vi "App Directory Folder and File Handler.vi"(8 "error in":errorcluster) -> (0 "error out":errorcluster, 1 "Setup Files Folder":path, 3 "Report Template Folder":path, 4 "Report Folder":path)   [LabVIEW 2018, in "File IO.lvlib"]
uses:
  File IO.lvlib
  <vilib>/Utility/sysdir.llb/System Directory Type.ctl
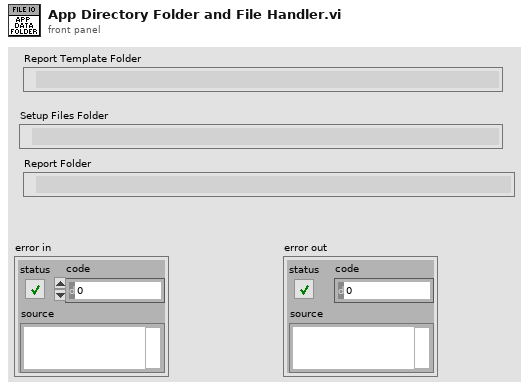
[diagram p1: front panel]
types:
  T1 = typedef "System Directory Type.ctl" = i32
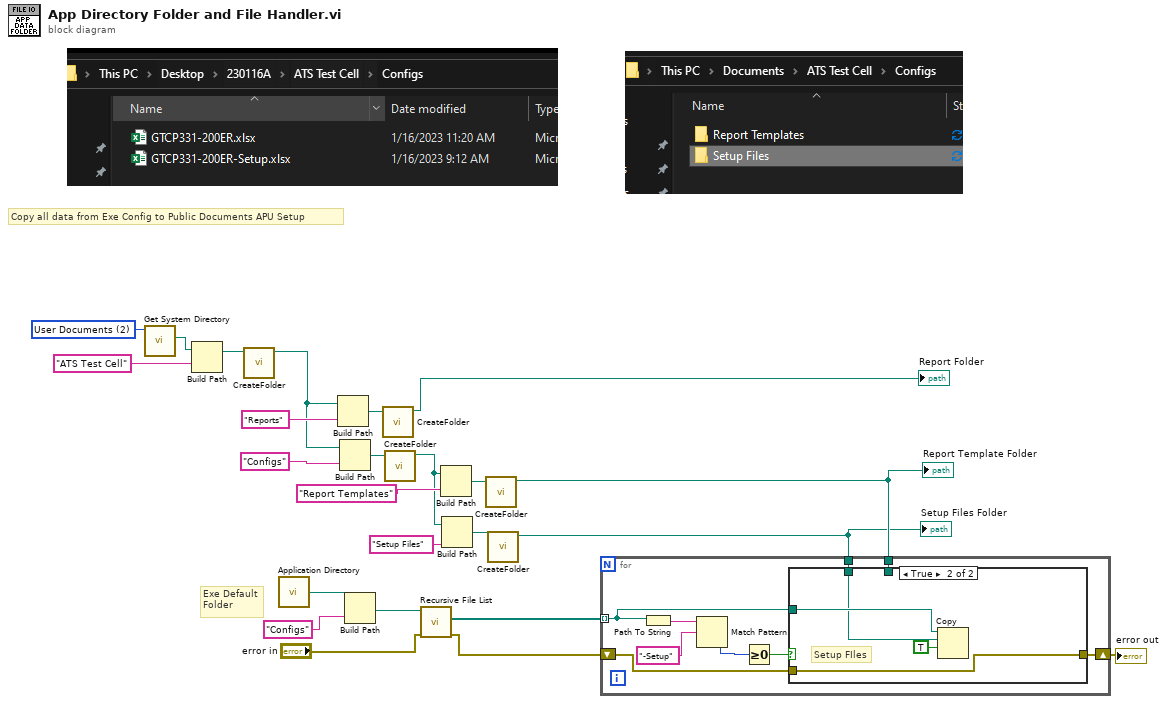
[diagram p0: block diagram]
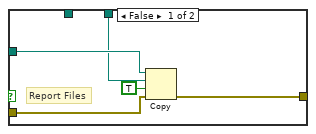
[diagram p2: hidden frame]
diagram:
  w24 = T1 2 items=["User Home"=0, "User Desktop"=1, "User Documents"=2, "User Application Data"=3, "User Preferences"=4, "User Temporary"=5, "Public Documents"=6, "Public Application Data"=7, "Public Preferences"=8, "Public Cache"=13, "System Core Libraries"=9, "System Installed Libraries"=10, "Application Files"=11, "Boot Volume Root"=12] ("system directory type")
  # "Exe Default\nFolder"
  # "Copy all data from Exe Config to Public Documents APU Setup"
  n1 = call <vilib>:"Get System Directory.vi"("system directory type"=w24) -> ("system directory"=w23:path)  [unwired: 10 in]
  n2 = Build Path(base path=w23, name or relative path="ATS Test Cell") -> (appended path=w15:path)
  n3 = call "CreateFolder.vi"("appended path"=w15) -> ("dup path"=w14:path)  [unwired: 9 in, 1 out]
  n4 = call <vilib>:"Application Directory.vi"() -> ("Application Directory"=w20:path)
  n5 = Build Path(base path=w14, name or relative path="Reports") -> (appended path=w18:path)
  n6 = Build Path(base path=w14, name or relative path="Configs") -> (appended path=w17:path)
  n7 = Build Path(base path=w20, name or relative path="Configs") -> (appended path=w7:path)
  n8 = call "CreateFolder.vi"("appended path"=w18) -> ("dup path"=→"Report Folder":path)  [unwired: 9 in, 1 out]
  n9 = call "CreateFolder.vi"("appended path"=w17) -> ("dup path"=w10:path)  [unwired: 9 in, 1 out]
  n10 = call <vilib>:"Recursive File List.vi"("error in (no error)"="error in", "Folder Path"=w7) -> ("error out"=w2:errorcluster, "All Files in Dir"=w6:path[])  [unwired: 5 in, 3 out]
  n11 = Build Path(base path=w10, name or relative path="Report Templates") -> (appended path=w13:path)
  n12 = Build Path(base path=w10, name or relative path="Setup Files") -> (appended path=w11:path)
  n13 = call "CreateFolder.vi"("appended path"=w13) -> ("dup path"=w5:path)  [unwired: 9 in, 1 out]
  "Report Template Folder" <- w5
  n14 = call "CreateFolder.vi"("appended path"=w11) -> ("dup path"=w4:path)  [unwired: 9 in, 1 out]
  "Setup Files Folder" <- w4
  n15 = for {
    tunnel: w6 -> [w29] mode=indexing
    tunnel: w4 -> [w28]
    tunnel: w5 -> [w27]
    shift-right: [w25] -> w1
    shift-left: w2 -> [w26]
    n16 = Path To String(path=w29) -> (string=w33:string)
    n17 = Match Pattern(string=w33, regular expression="-Setup") -> (offset past match=w31:i32)  [unwired: 1 in, 3 out]
    n18 = Greater Or Equal To 0?(x=w31) -> (x >= 0?=w30:bool)
    n19 = case shown="True" w30 {
      tunnel: w29 -> [w37 w41]
      tunnel: w28 -> [_ w40]
      tunnel: w27 -> [w36 _]
      tunnel: w26 -> [w35 w39]
      tunnel: [w34 w39] -> w25
      frame False {
        # "Report Files"
        n20 = Copy(8:w35, 9:TRUE ("overwrite (F)"), 10:w36, 11:w37) -> (0:w34:errorcluster)  [unwired: 1 in, 2 out]
      }
      frame True {
        # "Setup FIles"
        n21 = Copy(9:TRUE ("overwrite (F)"), 10:w40, 11:w41) -> ()  [unwired: 2 in, 3 out]
      }
    }
  }
  "error out" <- w1
